vi "sonarSetLights.vi"(0 "error in":errorcluster, 2 "Lights":T1, 3 "node":string) -> (1 "error out":errorcluster)   [LabVIEW 2015]
uses:
  ROS/Code/Console/Servers/ServerSubs/TopicDef.ctl
  ROS/Code/SubVIs/_ROSDirection.ctl
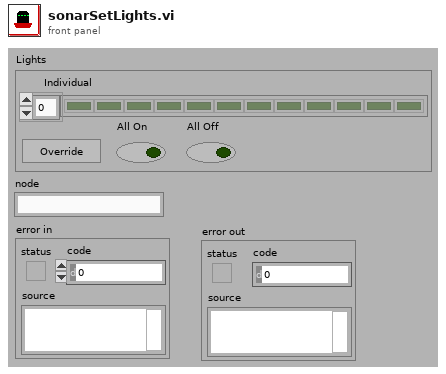
[diagram p1: front panel]
types:
  T1 = cluster{"Behavior":bool, "All On":bool, "All Off":bool, "Individual":bool[]}
  T2 = typedef "TopicDef.ctl" = cluster{"Topic":string, "Type":string, "Action":T3, "Update (ms)":u16, "queue size":u16}
  T3 = typedef "_ROSDirection.ctl" = enum16{"Node", "Publisher", "Subscriber", "ServiceClient", "ServiceProvider"}
  T4 = typedef "_ROSControl.ctl" = cluster{"topic port":u16, "Node":string, "topic":string, "type":string, "node port":u16, "error ":errorcluster, "Direction":T3, "Update (ms)":u16, "FIFO size":u16}
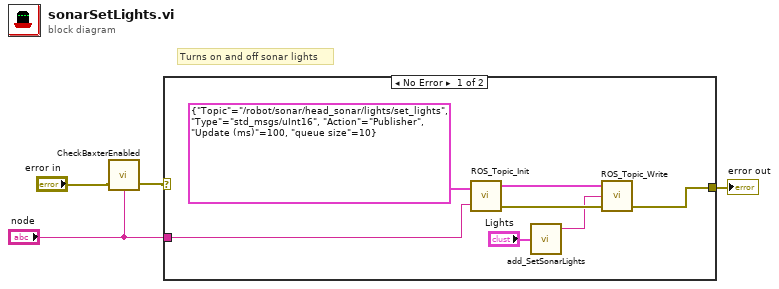
[diagram p0: block diagram]
diagram:
  # "Turns on and off sonar lights"
  n1 = call "CheckBaxterEnabled.vi"("error in"="error in", "node"="node") -> ("error out"=w2:errorcluster)  [unwired: 2 in]
  n2 = case shown="No Error" w2 {
    selector: w2 -> [_ w12]
    tunnel: [w5 w12] -> w4
    tunnel: "node" -> [w8 _]
    frame No Error {
      n3 = call "ROS_Topic_Init.vi"("Definitions"=T2 {"Topic"="/robot/sonar/head_sonar/lights/set_lights", "Type"="std_msgs/uInt16", "Action"=enum."Publisher", "Update (ms)"=100, "queue size"=10}, "node"=w8) -> ("ROS out"=w11:T4, "error out"=w7:errorcluster)  [unwired: 1 in]
      n4 = call "add_SetSonarLights.vi"("Lights"="Lights") -> ("msg out"=w6:string)  [unwired: 4 in]
      n5 = call "ROS_Topic_Write.vi"("error in (no error)"=w7, "Msg in"=w6, "ROS in"=w11) -> ("error out"=w5:errorcluster)  [unwired: 1 in, 1 out]
    }
    frame Error {
    }
  }
  "error out" <- w4
